vi "Zeitstempel letzte Kalibrierungen.vi"(6 "Aktionen":T1) -> (2 "Zeitstempeln":timestamp[](array[timestamp]) format="%<%H:%M:%S\n%x>T")   [LabVIEW 2020, in "FT-IR.lvlib"]
uses:
  FT-IR.lvlib
  Aktionen Zeitstempel speichern.ctl
  Allgemein/allgemeine Sub-VIs.lvlib
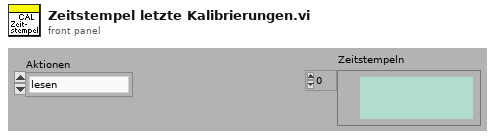
[diagram p1: front panel]
types:
  T1 = typedef "FT-IR.lvlib/Aktionen Zeitstempel speichern.ctl" = enum16{"lesen", "Zeitstempel NEU", "laden", "speichern"}
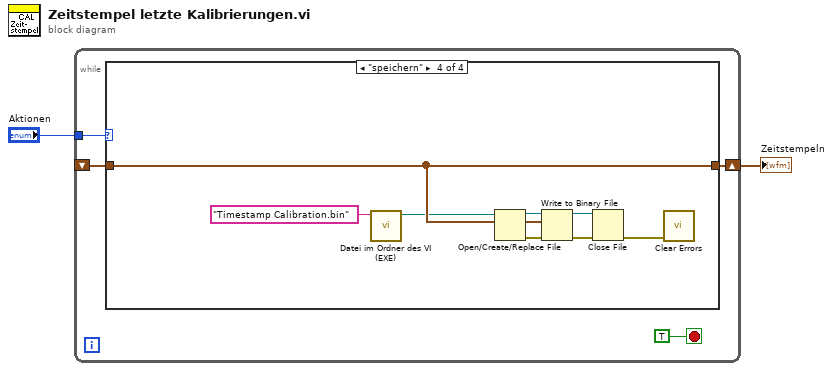
[diagram p0: block diagram]
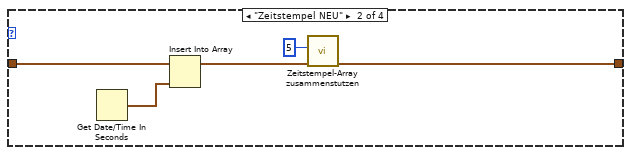
[diagram p3: hidden frame]
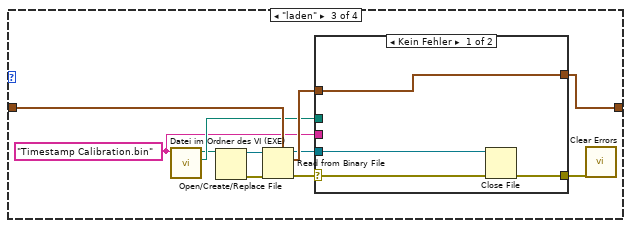
[diagram p4: hidden frame]
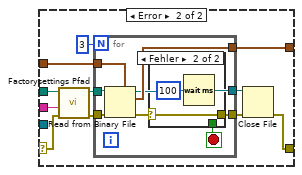
[diagram p5: hidden frame]
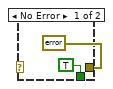
[diagram p6: hidden frame]
diagram:
  n1 = while {
    tunnel: "Aktionen" -> [w5]
    shift-right: [w4] -> w2
    shift-left: _ -> [w3]
    stop <- TRUE stop-if-true
    n2 = case shown="\"speichern\"" w5 {
      tunnel: [w7 w9 w21 w58] -> w4
      tunnel: w3 -> [w7 w11 w23 w58]
      frame "lesen", Default {
      }
      frame "Zeitstempel NEU" {
        n3 = Get Date/Time In Seconds() -> (seconds since 1Jan1904=w12:timestamp)
        n4 = Insert Into Array(array=w11, new element=w12) -> (w10:timestamp[])  [unwired: 1 in]
        n5 = call "Zeitstempel-Array zusammenstutzen.vi"("Array"=w10, "Anzahl Elemente"=5) -> ("Array"=w9:timestamp[])  [unwired: 9 in]
      }
      frame "laden" {
        w17 = "Timestamp Calibration.bin" ("Dateiname")
        n6 = call "Datei im Ordner des VI (EXE).vi"("Dateiname"=w17) -> ("Ordner des Haupt-VIs"=w20:path, "Dateipfad im Ordner des Haupt-VIs"=w14:path)  [unwired: 8 in, 1 out]
        n7 = Open/Create/Replace File(file path (use dialog)=w14) -> (refnum out=w13:refnum<file>, error out=w15:errorcluster)  [unwired: 5 in, 1 out]
        n8 = Read from Binary File(5:w23, 8:w15, 11:w13) -> (0:w19:errorcluster, 2:w22:timestamp[], 3:w18:refnum<file>)  [unwired: 4 out]
        n9 = case shown="Kein Fehler" w19 {
          selector: w19 -> [w26 w30]
          tunnel: w20 -> [_ w31]
          tunnel: w22 -> [w27 w29]
          tunnel: [w27 w37] -> w21
          tunnel: [w24 w35] -> w16
          tunnel: w18 -> [w25 _]
          tunnel: w17 -> [_ w28]
          frame No Error {
            n10 = Close File(refnum=w25, error in=w26) -> (error out=w24:errorcluster)  [unwired: 1 out]
          }
          frame Error {
            n11 = call "Factorysettings Pfad.vi"("error in (no error)"=w30, "Dateiname"=w28, "Ordner des Haupt-VIs"=w31) -> ("error out"=w32:errorcluster, "Pfad Factorysettings"=w33:path)  [unwired: 7 in]
            n12 = for {
              N: 3 -> [_]
              tunnel: w32 -> [w44]
              tunnel: w33 -> [w43]
              tunnel: [w42] -> w37
              tunnel: [w41] -> w36
              tunnel: [w40] -> w34
              tunnel: w29 -> [w39]
              stop <- w45 stop-if-true
              n13 = Read from Binary File(5:w39, 8:w44, 11:w43) -> (0:w46:errorcluster, 2:w42:timestamp[], 3:w40:refnum<file>)  [unwired: 3 in, 1 out]
              n14 = case shown="Fehler" w46 {
                selector: w46 -> [_ w49]
                tunnel: [TRUE _] -> w45
                tunnel: [errorcluster {"status"=FALSE, "code"=0, "source"=""} ("error IO") w49] -> w41
                frame No Error {
                }
                frame Error {
                  n15 = Wait (ms)(milliseconds to wait=u32 100 ("Zu wartende ms")) -> ()  [unwired: 1 out]
                }
              }
            }
            n16 = Close File(refnum=w34, error in=w36) -> (error out=w35:errorcluster)  [unwired: 1 out]
          }
        }
        n17 = call <vilib>:"Clear Errors.vi"("error in (no error)"=w16) -> ()  [unwired: 5 in, 2 out]
      }
      frame "speichern" {
        n18 = call "Datei im Ordner des VI (EXE).vi"("Dateiname"="Timestamp Calibration.bin") -> ("Dateipfad im Ordner des Haupt-VIs"=w56:path)  [unwired: 8 in, 2 out]
        n19 = Open/Create/Replace File(file path (use dialog)=w56) -> (refnum out=w55:refnum<file>, error out=w54:errorcluster)  [unwired: 5 in, 1 out]
        n20 = Write to Binary File(file (use dialog)=w55, data=w58, error in=w54) -> (refnum out=w52:refnum<file>, error out=w53:errorcluster)  [unwired: 4 out]
        n21 = Close File(refnum=w52, error in=w53) -> (error out=w51:errorcluster)  [unwired: 1 out]
        n22 = call <vilib>:"Clear Errors.vi"("error in (no error)"=w51) -> ()  [unwired: 5 in, 2 out]
      }
    }
  }
  "Zeitstempeln" <- w2
